vi "Test_uart_01.vi"() -> ()   [LabVIEW 2025]
uses:
  <vilib>/Instr/_visa.llb/VISA Configure Serial Port (Instr).vi
panel:
  in  "Tab Control":enum32{"CONTROL DE MOTOR (RMP's y ARX)"}(tab)
  in  "Stop Button":bool
  in  "CAJA ENGRANES":sgl
  out "Waveform Chart":cluster{"Número":sgl, "Número":sgl}(graph)
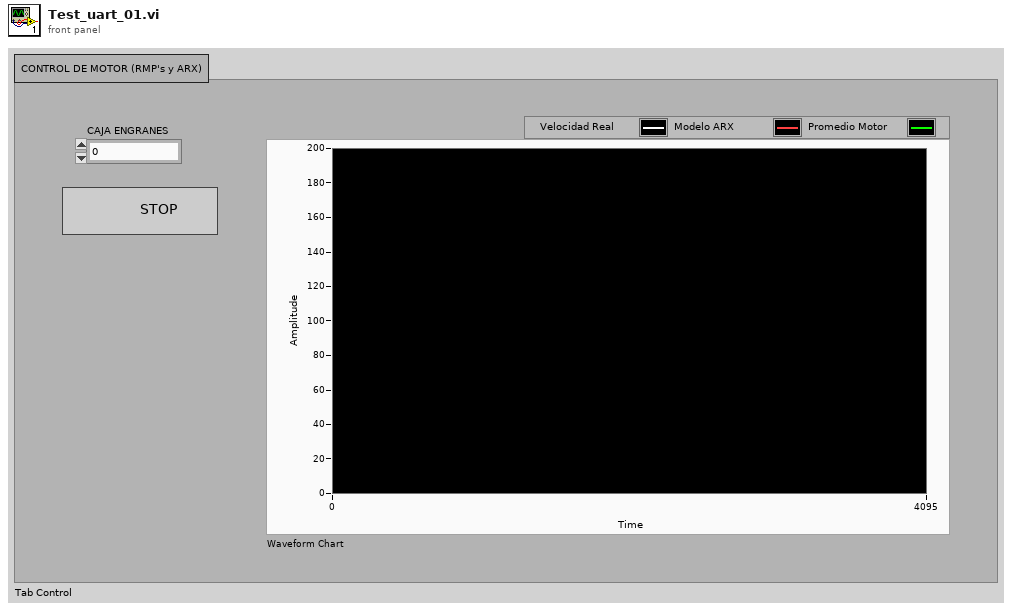
[diagram p1: front panel]
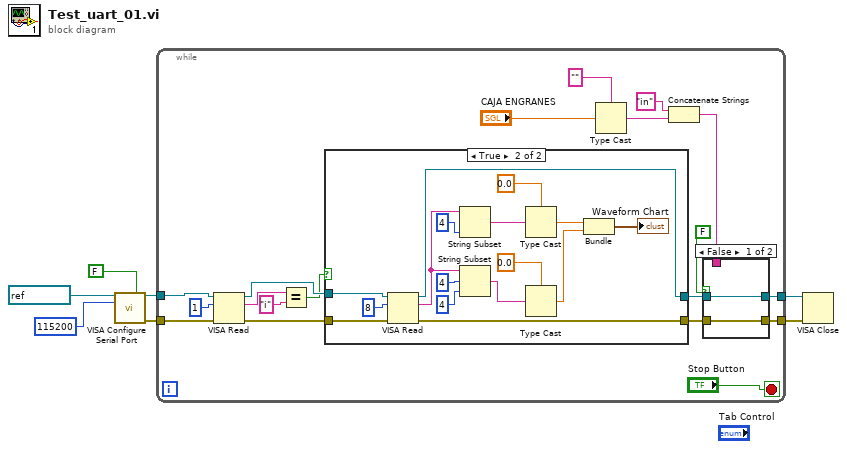
[diagram p0: block diagram]
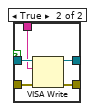
[diagram p2: hidden frame]
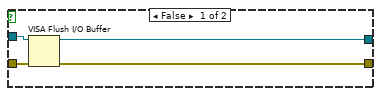
[diagram p3: hidden frame]
diagram:
  n1 = call-poly "VISA Configure Serial Port"("VISA resource name"=refnum<visa-resource-name> "COM4", "Enable Termination\nChar (T)"=FALSE ("Enable Termination\nChar (T)"), "baud rate (9600)"=u32 115200) -> ("VISA resource name out"=w2:refnum<visa-resource-name>, "error out"=w1:errorcluster)  [unwired: 11 in]
  n2 = while {
    tunnel: w2 -> [w24]
    tunnel: w1 -> [w23]
    tunnel: [w14] -> w7
    tunnel: [w15] -> w6
    stop <- "Stop Button" stop-if-true
    n3 = VISA Read(VISA resource name=w24, byte count=u32 1, error in (no error)=w23) -> (VISA resource name out=w22:refnum<visa-resource-name>, read buffer=w20:string, error out=w21:errorcluster)  [unwired: 1 out]
    n4 = Equal?(x=w20, y="i") -> (x = y?=w18:bool)
    n5 = case shown="True" w18 {
      tunnel: [w37 w53] -> w13
      tunnel: [w36 w52] -> w12
      tunnel: w22 -> [w35 w49]
      tunnel: w21 -> [w34 w48]
      frame False {
        n6 = VISA Flush I/O Buffer(VISA resource name=w35, error in (no error)=w34) -> (VISA resource name out=w37:refnum<visa-resource-name>, error out=w36:errorcluster)  [unwired: 1 in]
      }
      frame True {
        n7 = VISA Read(VISA resource name=w49, byte count=u32 8, error in (no error)=w48) -> (VISA resource name out=w53:refnum<visa-resource-name>, read buffer=w44:string, error out=w52:errorcluster)  [unwired: 1 out]
        n8 = String Subset(string=w44, length (rest)=4 ("length (rest)")) -> (substring=w46:string)  [unwired: 1 in]
        n9 = String Subset(string=w44, offset (0)=4, length (rest)=4 ("length (rest)")) -> (substring=w38:string)
        n10 = Type Cast(type=sgl 0.0 ("Número"), x=w46) -> (*(type *) &x=w42:sgl)
        n11 = Type Cast(type=sgl 0.0 ("Número"), x=w38) -> (*(type *) &x=w39:sgl)
        n12 = Bundle("Número"=w42, "Número"=w39) -> (→"Waveform Chart":cluster{"Número":sgl, "Número":sgl})  [unwired: 1 in]
      }
    }
    n13 = Type Cast(type="", x="CAJA ENGRANES") -> (*(type *) &x=w10:string)
    n14 = Concatenate Strings("in", w10) -> (w9:string)
    n15 = case shown="False" FALSE {
      tunnel: [w27 w33] -> w15
      tunnel: [w28 w32] -> w14
      tunnel: w13 -> [w28 w31]
      tunnel: w12 -> [w27 w30]
      tunnel: w9 -> [_ w29]
      frame False {
      }
      frame True {
        n16 = VISA Write(VISA resource name=w31, write buffer=w29, error in (no error)=w30) -> (VISA resource name out=w32:refnum<visa-resource-name>, error out=w33:errorcluster)  [unwired: 1 out]
      }
    }
  }
  n17 = VISA Close(VISA resource name=w7, error in (no error)=w6) -> ()  [unwired: 1 out]
